vi "SimulatorLoop.vi"() -> ()   [LabVIEW 2016]
panel:
  out "output array":u64[](array[numeric])
  out "element 2":u64
  out "element":u64
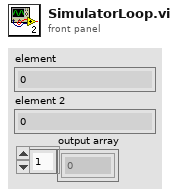
[diagram p1: front panel]
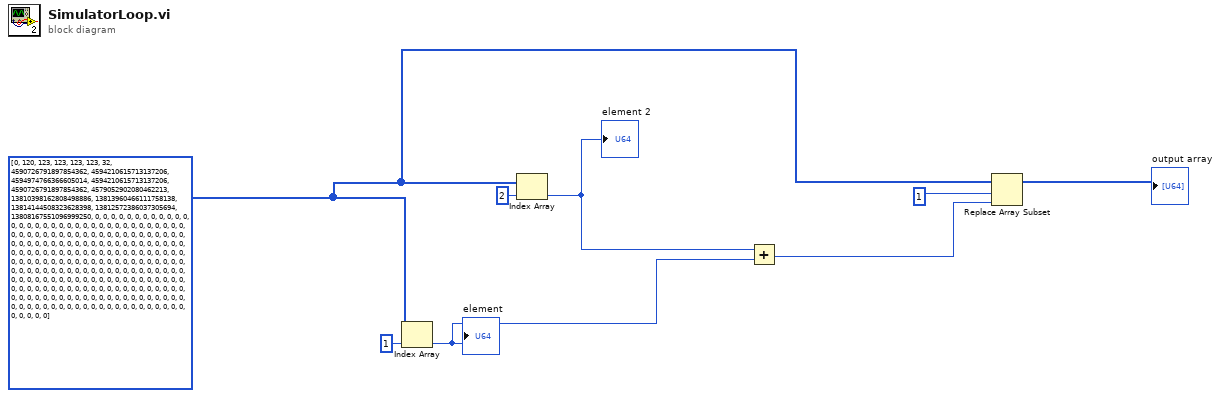
[diagram p0: block diagram]
diagram:
  w8 = u64[] [0, 120, 123, 123, 123, 123, 32, 4590726791897854362, 4594210615713137206, 4594974766366605014, 4594210615713137206, 4590726791897854362, 4579052902080462213, 13810398162808498886, 13813960466111758138, 13814144508323628398, 13812572386037305694, 13808167551096999250, 0, 0, 0, 0, 0, 0, 0, 0, 0, 0, 0, 0, 0, 0, 0, 0, 0, 0, 0, 0, 0, 0, 0, 0, 0, 0, 0, 0, 0, 0, 0, 0, 0, 0, 0, 0, 0, 0, 0, 0, 0, 0, 0, 0, 0, 0, 0, 0, 0, 0, 0, 0, 0, 0, 0, 0, 0, 0, 0, 0, 0, 0, 0, 0, 0, 0, 0, 0, 0, 0, 0, 0, 0, 0, 0, 0, 0, 0, 0, 0, 0, 0, 0, 0, 0, 0, 0, 0, 0, 0, 0, 0, 0, 0, 0, 0, 0, 0, 0, 0, 0, 0, 0, 0, 0, 0, 0, 0, 0, 0, 0, 0, 0, 0, 0, 0, 0, 0, 0, 0, 0, 0, 0, 0, 0, 0, 0, 0, 0, 0, 0, 0, 0, 0, 0, 0, 0, 0, 0, 0, 0, 0, 0, 0, 0, 0, 0, 0, 0, 0, 0, 0, 0, 0, 0, 0, 0, 0, 0, 0, 0, 0, 0, 0, 0, 0, 0, 0, 0, 0, 0, 0, 0, 0, 0, 0, 0, 0, 0, 0, 0, 0, 0, 0, 0, 0, 0, 0, 0, 0, 0, 0, 0, 0, 0, 0, 0, 0, 0, 0, 0, 0, 0, 0, 0, 0, 0, 0, 0, 0, 0, 0, 0, 0, 0, 0, 0, 0, 0, 0, 0, 0, 0, 0, 0, 0, 0, 0, 0, 0, 0, 0, 0, 0, 0, 0, 0] ("DataMemory/Fxp")
  n1 = Index Array "Index Array"(array=w8, index=1) -> (element=w3:u64)
  "element" <- w3
  n2 = Index Array "Index Array"(array=w8, index=2) -> (element=w4:u64)
  "element 2" <- w4
  n3 = Add(x=w4, y=w3) -> (x+y=w2:u64)
  n4 = Replace Array Subset "Replace Array Subset"(array=w8, new element=w2, index=1) -> (→"output array":u64[])
